vi "FFT_Analysis.vi"(8 "Length of Sample":i32, 9 "Data":dbl[](array[numeric]), 10 "T_vect":dbl) -> (0 "Magnitude":dbl[](array[numeric]), 1 "Phase":dbl[](array[numeric]), 2 "Peaks":dbl[][](array[numeric]), 3 "XY Graph":cluster{"Y":dbl[], "Y":dbl[]}[](graph))   [LabVIEW 2018]
uses:
  <vilib>/Analysis/2dsp.llb/Real FFT.vi
  <vilib>/Analysis/NI_AALPro.lvlib
  <vilib>/ptbypt/NI_PtbyPt.lvlib
  <vilib>/Analysis/NI_AAL_SigProc.lvlib
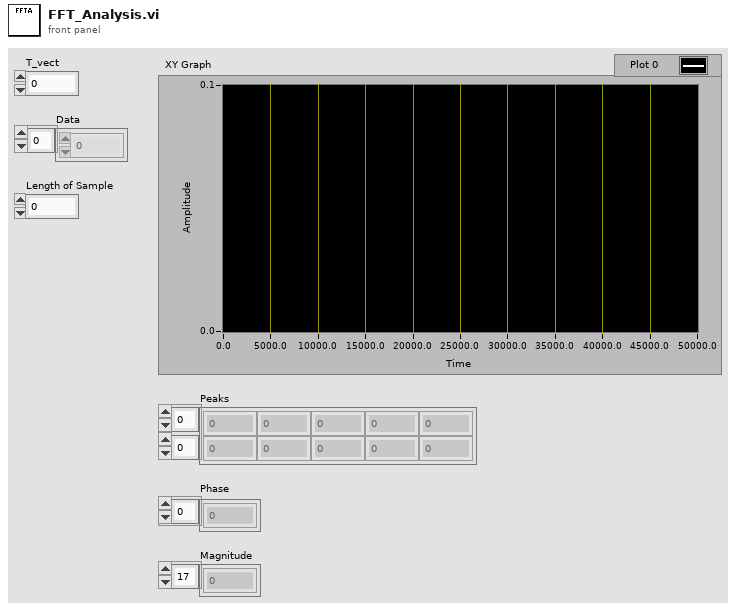
[diagram p1: front panel]
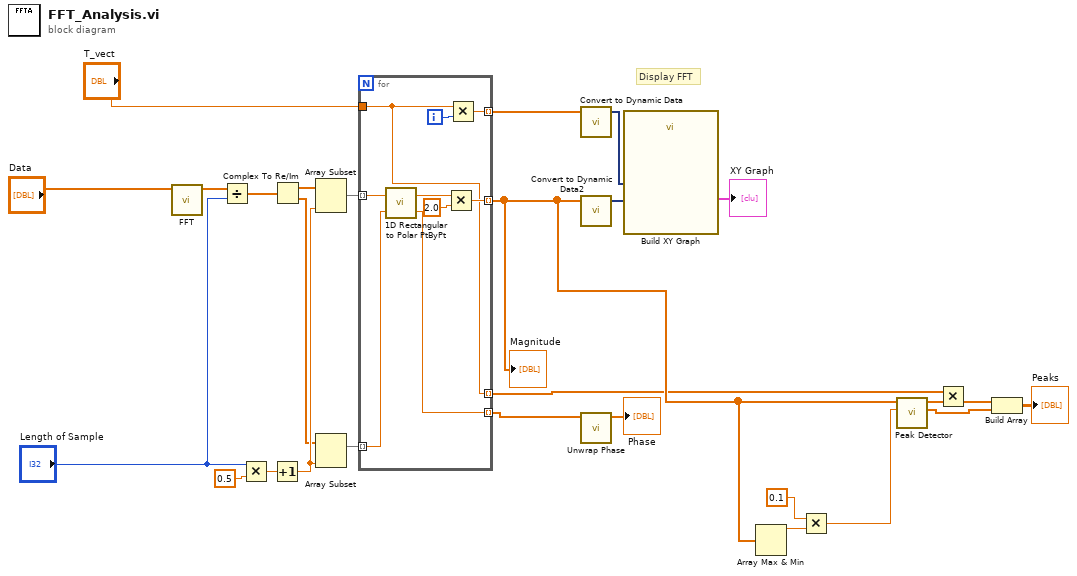
[diagram p0: block diagram]
diagram:
  # "Display FFT"
  n1 = call-poly <vilib>:"FFT.vi"("X"="Data") -> ("FFT {X}"=w16:cdb[])  [unwired: 9 in, 1 out]
  n2 = Divide(x=w16, y="Length of Sample") -> (x/y=w7:cdb[])
  n3 = Multiply(x="Length of Sample", y=0.5) -> (x*y=w3:dbl)
  n4 = Increment(x=w3) -> (x+1=w14:dbl)
  n5 = Complex To Re/Im(x + iy=w7) -> (x=w1:dbl[], y=w4:dbl[])
  n6 = Array Subset(array=w1, length=w14) -> (w5:dbl[])  [unwired: 1 in]
  n7 = Array Subset(array=w4, length=w14) -> (w6:dbl[])  [unwired: 1 in]
  n8 = for {
    tunnel: w5 -> [w36] mode=indexing
    tunnel: w6 -> [w35] mode=indexing
    tunnel: [w32] -> w22 mode=indexing
    tunnel: [w31] -> w9 mode=indexing
    tunnel: "T_vect" -> [w28]
    tunnel: [w30] -> w15 mode=indexing
    tunnel: [w28] -> w19 mode=indexing
    i -> [w29]
    n9 = call <vilib>:"1D Rectangular to Polar PtByPt.vi"("y"=w35, "x"=w36) -> ("phase"=w31:dbl, "magnitude"=w34:dbl)
    n10 = Multiply(x=w34, y=2.0) -> (x*y=w32:dbl)
    n11 = Multiply(x=w28, y=w29) -> (x*y=w30:dbl)
  }
  "Magnitude" <- w22
  n12 = call "Convert to Dynamic Data"("Array"=w15) -> ("Dynamic Data Type"=w12:dynamicdata)  [unwired: 3 in]
  n13 = call "Convert to Dynamic Data2"("Array"=w22) -> ("Dynamic Data Type"=w13:dynamicdata)  [unwired: 3 in]
  n14 = call <vilib>:"Unwrap Phase.vi"("Phase"=w9) -> ("Unwrapped Phase"=→"Phase":dbl[])  [unwired: 9 in, 1 out]
  n15 = call "Build XY Graph"("Y Input"=w13, "X Input"=w12) -> ("XY Graph"=→"XY Graph":cluster{"X":dbl[], "Y":dbl[]}[])  [unwired: 8 in, 1 out]
  n16 = Array Max & Min(array=w22) -> (max value=w23:dbl)  [unwired: 3 out]
  n17 = Multiply(x=0.1 ("threshold"), y=w23) -> (x*y=w25:dbl)
  n18 = call <vilib>:"Peak Detector.vi"("threshold"=w25, "X"=w22) -> ("Amplitudes"=w20:dbl[], "Locations"=w17:dbl[])  [unwired: 5 in, 3 out]
  n19 = Multiply(x=w19, y=w17) -> (x*y=w18:dbl[])
  n20 = Build Array(w18, w20) -> (→"Peaks":dbl[][])
